vi "rqcAlice Modulator Window Configure.vi"(8 "error in":errorcluster, 10 "Modulator config":T1, 11 "Alice FPGA Reference In":refnum<k20>) -> (0 "error out":errorcluster, 3 "Alice FPGA Reference Out":refnum<k20>)   [LabVIEW 2019]
uses:
  FPGA/Alice/Custom Controls/Phase Modulator/rqcAlice Mod.Config.ctl
  <vilib>/Utility/error.llb/Error Cluster From Error Code.vi
  <vilib>/rvi/errors/niLvFpgaAdjustHostInterfaceError.vi
  <vilib>/rvi/interface/nirviReadWriteControl/nirviReadWriteControl.xnode
  NiFpgaLv.dll
  <vilib>/rvi/interface/Simulation/niFpgaSimulationCallBeginRW.vi
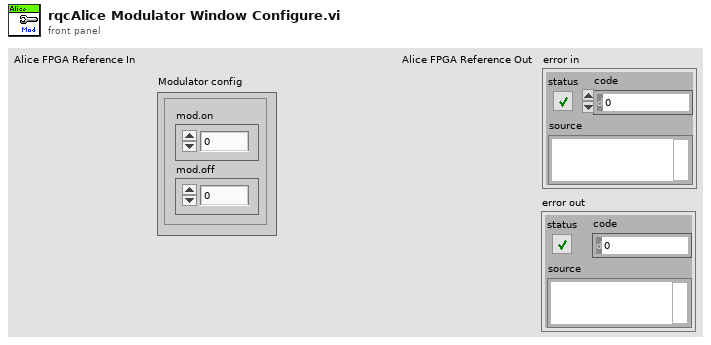
[diagram p1: front panel]
types:
  T1 = typedef "rqcAlice Mod.Config.ctl" = cluster{"mod.on":u8, "mod.off":u8}
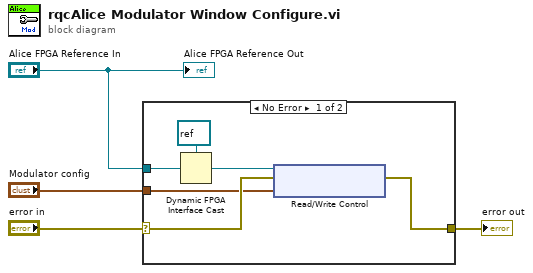
[diagram p0: block diagram]
diagram:
  n1 = case shown="No Error" "error in" {
    selector: "error in" -> [w7 w11]
    tunnel: [w6 w11] -> w3
    tunnel: "Alice FPGA Reference In" -> [w10 _]
    tunnel: "Modulator config" -> [w5 _]
    frame No Error {
      n2 = Dynamic FPGA Interface Cast(Session In=refnum<k20> refnum ("Type"), Type=w10) -> (Session Out=w8:refnum<k20>)
      n3 = xnode "Read/Write Control"("FPGA VI Reference In"=w8, "error in"=w7, "modulator.config"=w5) -> ("error out"=w6:errorcluster)  [unwired: 1 out]
    }
    frame Error {
    }
  }
  "error out" <- w3
  "Alice FPGA Reference Out" <- "Alice FPGA Reference In"
